vi "Swap Refs.vi"(8 "error in (no error)":errorcluster, 10 "Old Ref":refnum<class "Alicat.lvclass">, 11 "New Ref":refnum<class "P.lvclass">) -> (0 "error out":errorcluster, 3 "Alicat_P out":refnum<class "P.lvclass">)   [LabVIEW 2013, in "Alicat.lvlib" / "P.lvclass"]
uses:
  P.lvclass
  Alicat.lvclass
  Read formula_info.vi
  Write formula_info.vi
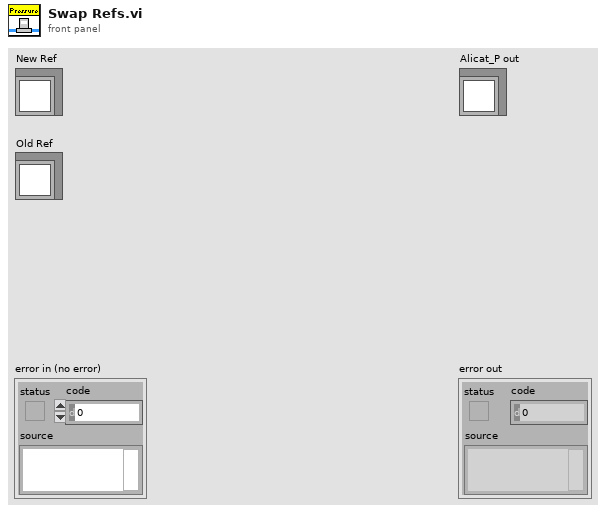
[diagram p1: front panel]
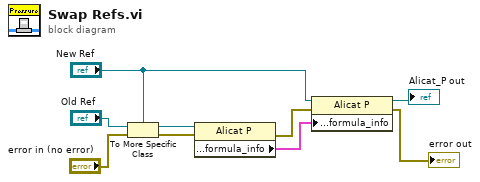
[diagram p0: block diagram]
diagram:
  n1 = To More Specific Class(target class="New Ref", reference="Old Ref", error in="error in (no error)") -> (specific class reference=w8:refnum<class "P.lvclass">, error out=w3:errorcluster)
  n2 = property class="Alicat P"(reference=w8, error in=w3) -> (error out=w5:errorcluster, "Data Access:formula_info"=w6:cluster{"Table":i32[][], "Y Values":dbl[]})  [unwired: 1 out]
  n3 = property class="Alicat P"(reference="New Ref", error in=w5, "Data Access:formula_info"=w6) -> (reference out=→"Alicat_P out":refnum<class "P.lvclass">, error out=→"error out":errorcluster)
